vi "SIMULATE.vi"(8 "error in (no error)":errorcluster, 11 "Stand in":refnum<class "Stand.lvclass">) -> (0 "error out":errorcluster, 3 "Stand out":refnum<class "Stand.lvclass">)   [LabVIEW 2019, in "Stand.lvclass"]
uses:
  Stand.lvclass
  Stand.lvclass/Stand.ctl
  FPGA_Interface_class/FPGA_Interface.lvclass
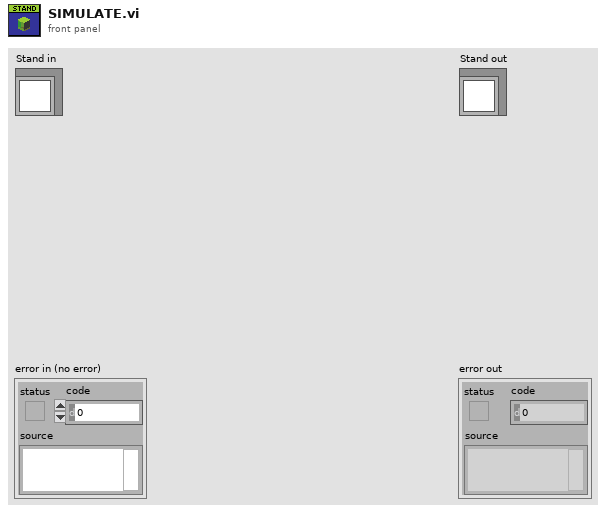
[diagram p1: front panel]
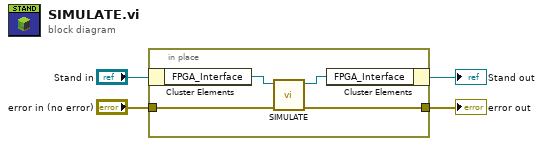
[diagram p0: block diagram]
diagram:
  n1 = in-place {
    in-place-border: "error in (no error)" -> [w6]
    in-place-border: [w5] -> w2
    n2 = in-place-cluster #1("Stand in") -> ("FPGA_Interface"=w8:refnum<class "FPGA_Interface.lvclass">)
    n3 = call-dynamic "SIMULATE.vi"("error in (no error)"=w6, "FPGA_Interface in"=w8) -> ("error out"=w5:errorcluster, "FPGA_Interface out"=w7:refnum<class "FPGA_Interface.lvclass">)  [unwired: 8 in]
    n4 = in-place-cluster #1("FPGA_Interface"=w7) -> (→"Stand out":refnum<class "Stand.lvclass">)
  }
  "error out" <- w2
